vi "Fit Transform.vi"(8 "error in (no error)":errorcluster caption="entrée d'erreur (pas d'erreur)", 10 "y":string[][](array[string]), 11 "MultiLabelBinarizer.lvclass":refnum<class "MultiLabelBinarizer.lvclass">) -> (0 "error out":errorcluster caption="sortie d'erreur", 2 "Data":T1, 3 "MultiLabelBinarizer.lvclass":refnum<class "MultiLabelBinarizer.lvclass">)   [LabVIEW 2020, in "MultiLabelBinarizer.lvclass"]
doc: "Fit the label sets binarizer and transform the given label sets. \n\nReturns : \n\n- y_indicator : array or CSR matrix, shape (n_samples, n_classes)\nA matrix such that y_indicator[i, j] = 1 iff classes_[j] is in y[i], and 0 otherwise."
uses:
  MultiLabelBinarizer.lvclass
  MultiLabelBinarizer.lvclass/MultiLabelBinarizer.ctl
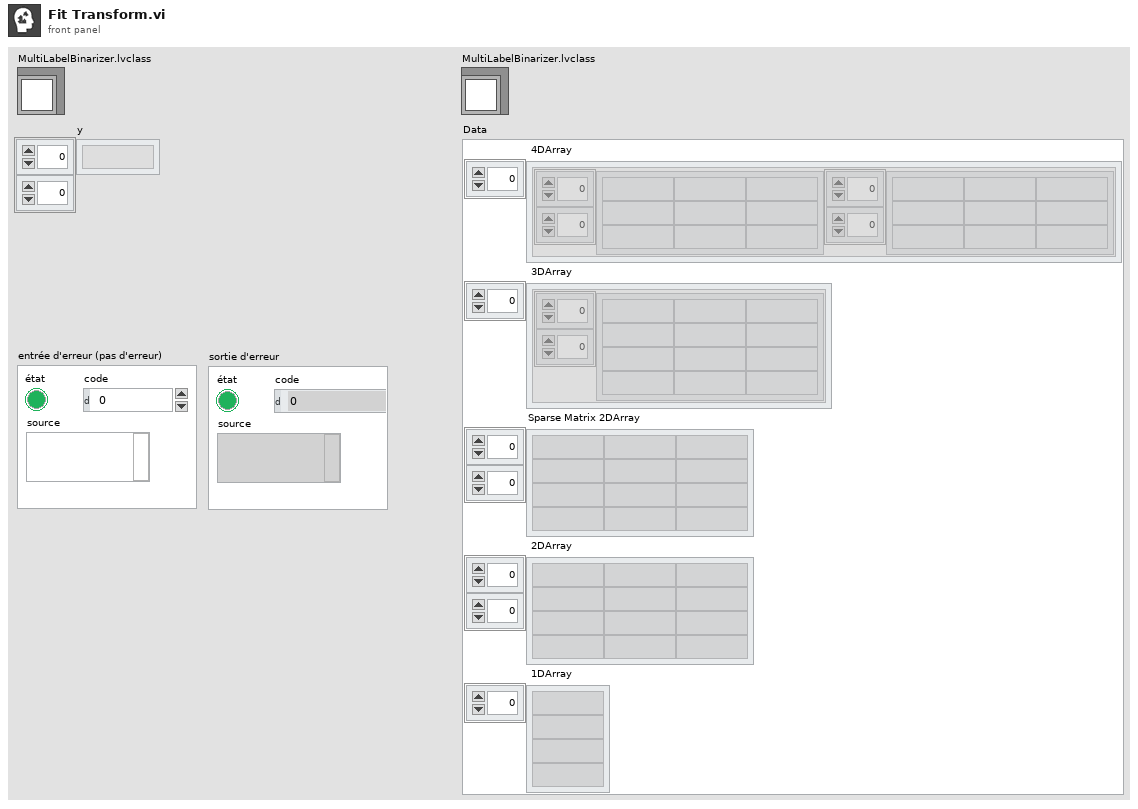
[diagram p1: front panel]
types:
  T1 = cluster{" 4DArray":cluster{"1":string[][], "2":string[][]}[], " 3DArray":cluster{"Tableau":string[][]}[], "Sparse Matrix 2DArray":string[][], " 2DArray":string[][], " 1DArray":string[]}
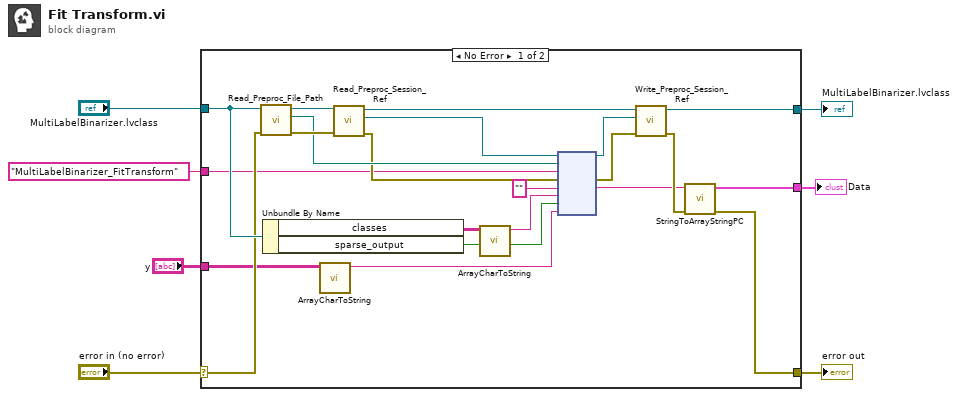
[diagram p0: block diagram]
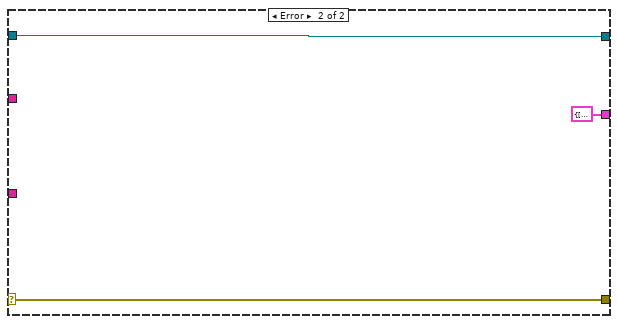
[diagram p2: hidden frame]
diagram:
  n1 = case shown="No Error" "error in (no error)" {
    selector: "error in (no error)" -> [w19 w32]
    tunnel: [w12 w32] -> w6
    tunnel: [w14 w31] -> w4
    tunnel: "MultiLabelBinarizer.lvclass" -> [w20 w31]
    tunnel: "MultiLabelBinarizer_FitTransform" ("Fonction") -> [w18 _]
    tunnel: [w13 T1 {" 4DArray"=[], " 3DArray"=[], "Sparse Matrix 2DArray"=[], " 2DArray"=[], " 1DArray"=[]} ("Data")] -> w2
    tunnel: "y" -> [w11 _]
    frame No Error {
      n2 = call-dynamic "Read_Preproc_File_Path.vi"("error in (no error)"=w19, "Python in"=w20) -> ("error out"=w28:errorcluster, "File_Path"=w25:path, "Python out"=w29:refnum<class "MultiLabelBinarizer.lvclass">)  [unwired: 7 in]
      n3 = Unbundle By Name(w20) -> ("classes"=w9:string[][], "sparse_output"=w17:bool)
      n4 = call "ArrayCharToString.vi"("TAB"=w11) -> ("Instruction"=w10:string)  [unwired: 10 in]
      n5 = call-dynamic "Read_Preproc_Session_Ref.vi"("error in (no error)"=w28, "Python in"=w29) -> ("error out"=w24:errorcluster, "Session_ref"=w26:refnum<k35>, "Python out"=w27:refnum<class "MultiLabelBinarizer.lvclass">)  [unwired: 7 in]
      n6 = call "ArrayCharToString.vi"("TAB"=w9) -> ("Instruction"=w8:string)  [unwired: 10 in]
      n7 = node(w26, w25, w18, w24, "", w8, w17, w10) -> (w22:refnum<k35>, w23:errorcluster, w15:string)  [unwired: 3 in, 2 out]
      n8 = call-dynamic "Write_Preproc_Session_Ref.vi"("error in (no error)"=w23, "Session_ref"=w22, "Python in"=w27) -> ("error out"=w16:errorcluster, "Python out"=w14:refnum<class "MultiLabelBinarizer.lvclass">)  [unwired: 7 in]
      n9 = call "StringToArrayStringPC.vi"("sortie d'erreur"=w16, "Return value"=w15) -> ("sortie d'erreur"=w12:errorcluster, "Data"=w13:T1)  [unwired: 8 in]
    }
    frame Error {
    }
  }
  "error out" <- w6
  "MultiLabelBinarizer.lvclass" <- w4
  "Data" <- w2
